vi "System@AddExternalDriver__Parameter.vi"(1 "ParamterIn":string) -> (0 "ParamterOut":string)   [LabVIEW 2019]
uses:
  MainFrame/Global.vi
panel:
  in  "Driver":string(combo)
  in  "Module":string(combo)
  in  "Confirm":bool
  # "System@AddExternalDriver $Module,$Driver\nModule Directory is at MainPath\\ExternalModules\\$Module\\$Driver"
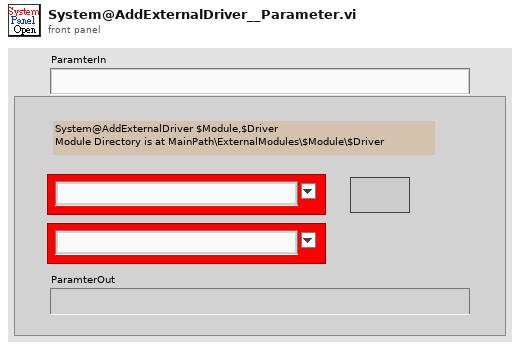
[diagram p1: front panel]
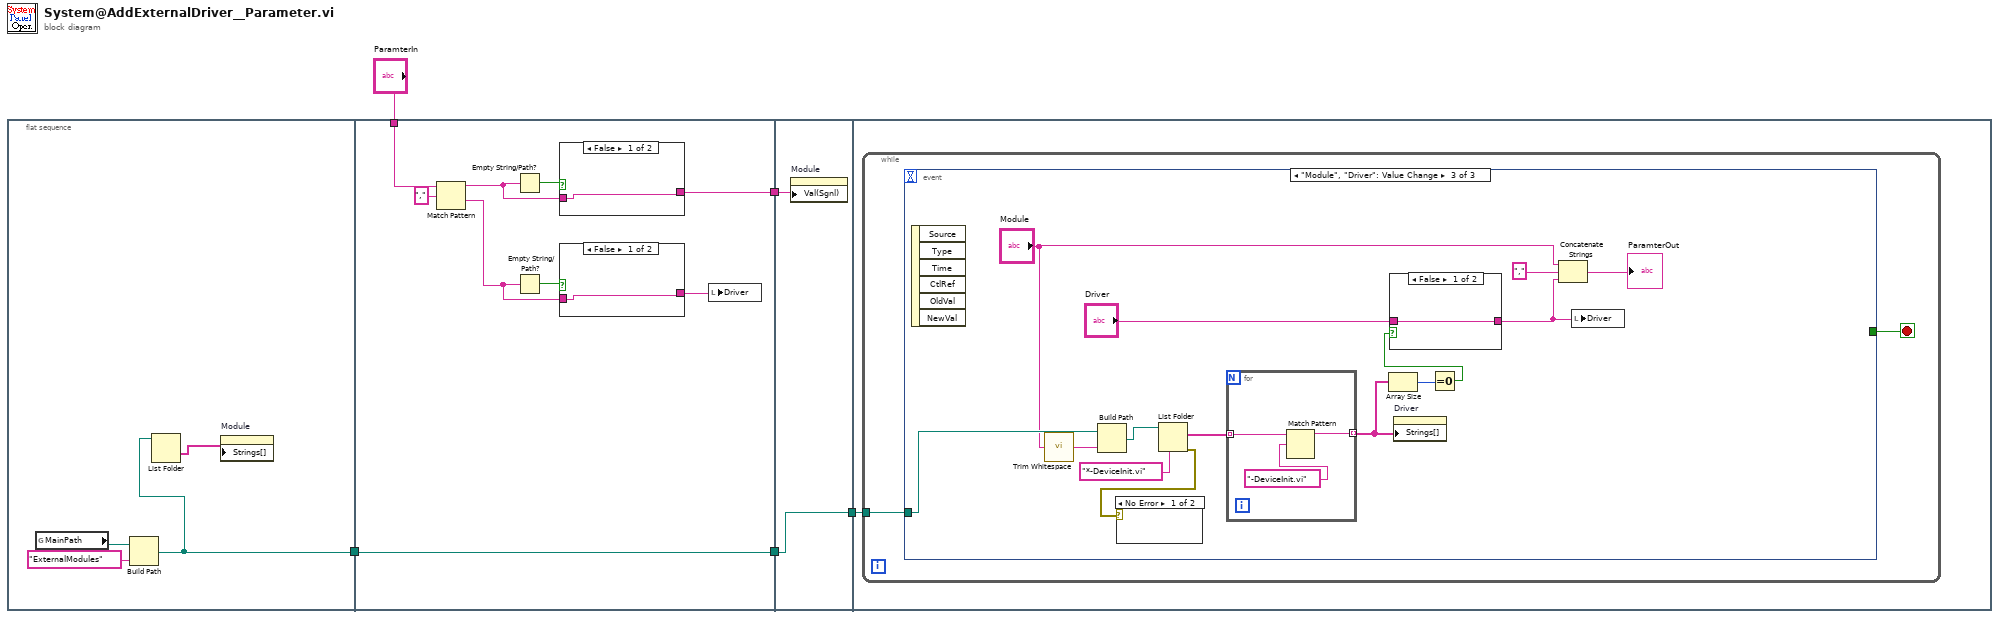
[diagram p0: block diagram]
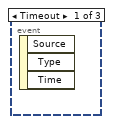
[diagram p4: hidden frame]
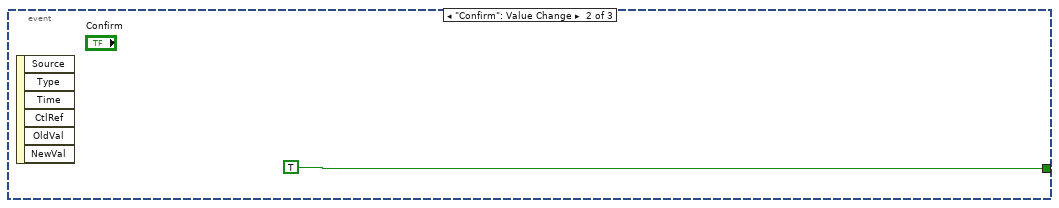
[diagram p5: hidden frame]
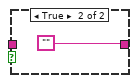
[diagram p7: hidden frame]
diagram:
  n1 = flat-sequence {
    tunnel: [w6] -> w2
    tunnel: "ParamterIn" -> [w16]
    tunnel: [w17] -> w4
    tunnel: [w10] -> w3
    tunnel: w2 -> [w10]
    tunnel: w4 -> [w24]
    tunnel: w3 -> [w23]
    tunnel: [w23] -> w1
    tunnel: w1 -> [w25]
    frame #0 {
      n2 = global read "Global.vi" "MainPath"() -> (w9:path)
      n3 = Build Path(base path=w9, name or relative path="ExternalModules") -> (appended path=w6:path)
      n4 = List Folder(path=w6) -> (folder names=w7:string[])  [unwired: 3 in, 3 out]
      n5 = property on="Module" class="CmbBox"("Strings[]"=w7) -> ()  [unwired: 2 in, 2 out]
    }
    frame #1 {
      n6 = Match Pattern(string=w16, regular expression=",") -> (before substring=w13:string, after substring=w12:string)  [unwired: 1 in, 2 out]
      n7 = Empty String/Path?(string/path=w13) -> (empty?=w18:bool)
      n8 = Empty String/Path?(string/path=w12) -> (empty?=w14:bool)
      n9 = case shown="False" w18 {
        tunnel: w13 -> [w21 w22]
        tunnel: [w21 w22] -> w17
        frame False {
        }
        frame True {
        }
      }
      n10 = case shown="False" w14 {
        tunnel: w12 -> [w19 w20]
        tunnel: [w19 w20] -> w11
        frame False {
        }
        frame True {
        }
      }
      n11 = local write "Driver"(w11) -> ()
    }
    frame #2 {
      n12 = property on="Module" class="CmbBox"("Val(Sgnl)"=w24) -> ()  [unwired: 2 in, 2 out]
    }
    frame #3 {
      n13 = while {
        tunnel: w25 -> [w26]
        stop <- w27 stop-if-true
        n14 = event shown="[2] \"Module\", \"Driver\": Value Change" {
          selector: _ -> [_ _ _]
          dyn-events: _ -> [_ _ _]
          timeout: _ -> [_ _ _]
          tunnel: [_ TRUE _] -> w27
          tunnel: w26 -> [_ _ w40]
          event Timeout {
            n15 = event-data() -> ()  [unwired: 1 in, 3 out]
          }
          event "Confirm": Value Change {
            n16 = event-data() -> ()  [unwired: 1 in, 6 out]
          }
          event "Module", "Driver": Value Change {
            n17 = event-data() -> ()  [unwired: 1 in, 6 out]
            n18 = call <vilib>:"Trim Whitespace.vi"("string"="Module") -> ("trimmed string"=w39:string)  [unwired: 1 in]
            n19 = Build Path(base path=w40, name or relative path=w39) -> (appended path=w37:path)
            n20 = List Folder(path=w37, pattern="*-DeviceInit.vi") -> (filenames=w35:string[], error out=w29:errorcluster)  [unwired: 2 in, 2 out]
            n21 = case shown="No Error" w29 {
              frame No Error {
              }
              frame Error {
              }
            }
            n22 = for {
              tunnel: w35 -> [w47] mode=indexing
              tunnel: [w45] -> w34 mode=indexing
              n23 = Match Pattern(string=w47, regular expression="-DeviceInit.vi" ("pattern")) -> (before substring=w45:string)  [unwired: 1 in, 3 out]
            }
            n24 = Array Size(array=w34) -> (size(s)=w33:i32)
            n25 = property on="Driver" class="CmbBox"("Strings[]"=w34) -> ()  [unwired: 2 in, 2 out]
            n26 = Equal To 0?(x=w33) -> (x = 0?=w32:bool)
            n27 = case shown="False" w32 {
              tunnel: [w43 ""] -> w30
              tunnel: "Driver" -> [w43 _]
              frame False {
              }
              frame True {
              }
            }
            n28 = Concatenate Strings("Module", "," ("string"), w30) -> (→"ParamterOut":string)
            n29 = local write "Driver"(w30) -> ()
          }
        }
      }
    }
  }
